vi "main.vi"() -> ()   [LabVIEW 2019]
uses:
  <instrlib>/Keithley 2600 Series/Keithley 2600 Series.lvlib
panel:
  in  "图数据":dbl[][](array[numeric])
  in  "自行输入":bool
  in  "时序优先":bool
  in  "维持时间(ms)":dbl=25.0
  in  "nplc":dbl=1.0
  in  "电压改变量":dbl=0.1 min=1e-05 max=0.1 step=1e-05
  in  "清除缓存数据":bool
  out "负时间标":timestamp
  out "正时间标":timestamp
  in  "正向状态":enum32{"SET", "RESET"}(radio)
  in  "测试人员":string
  in  "衬底":string(combo)
  in  "阻变物质":string(combo)
  in  "保存数据":bool
  out "负标记":bool
  out "正标记":bool
  out "XY图":picture
  in  "log":bool
  in  "负向扫描":bool
  in  "正向扫描":bool
  in  "反向扫描电压(V)":dbl=1.0 min=0.0 max=40.0 step=0.1
  in  "正向扫描电压(V)":dbl=1.0 min=0.0 max=40.0 step=0.1
  in  "反向极限电流(mA)":dbl=1.0 min=0.0 max=1000.0 step=0.1
  in  "正向极限电流(mA)":dbl=1.0 min=0.0 max=10.0 step=0.1
  in  "VISA resource name":refnum<visa-resource-name>
  in  "停止":bool
  in  "负":dbl[][](array[numeric])
  in  "正":dbl[][](array[numeric])
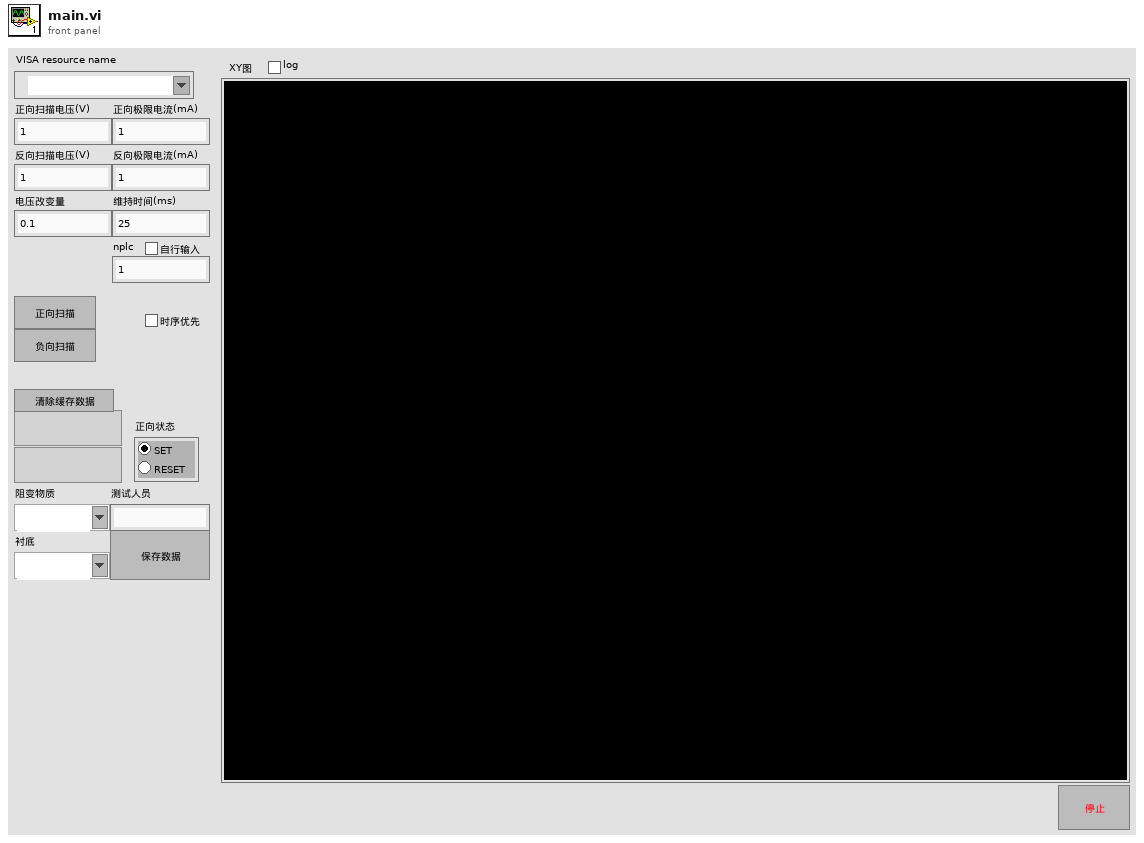
[diagram p1: front panel]
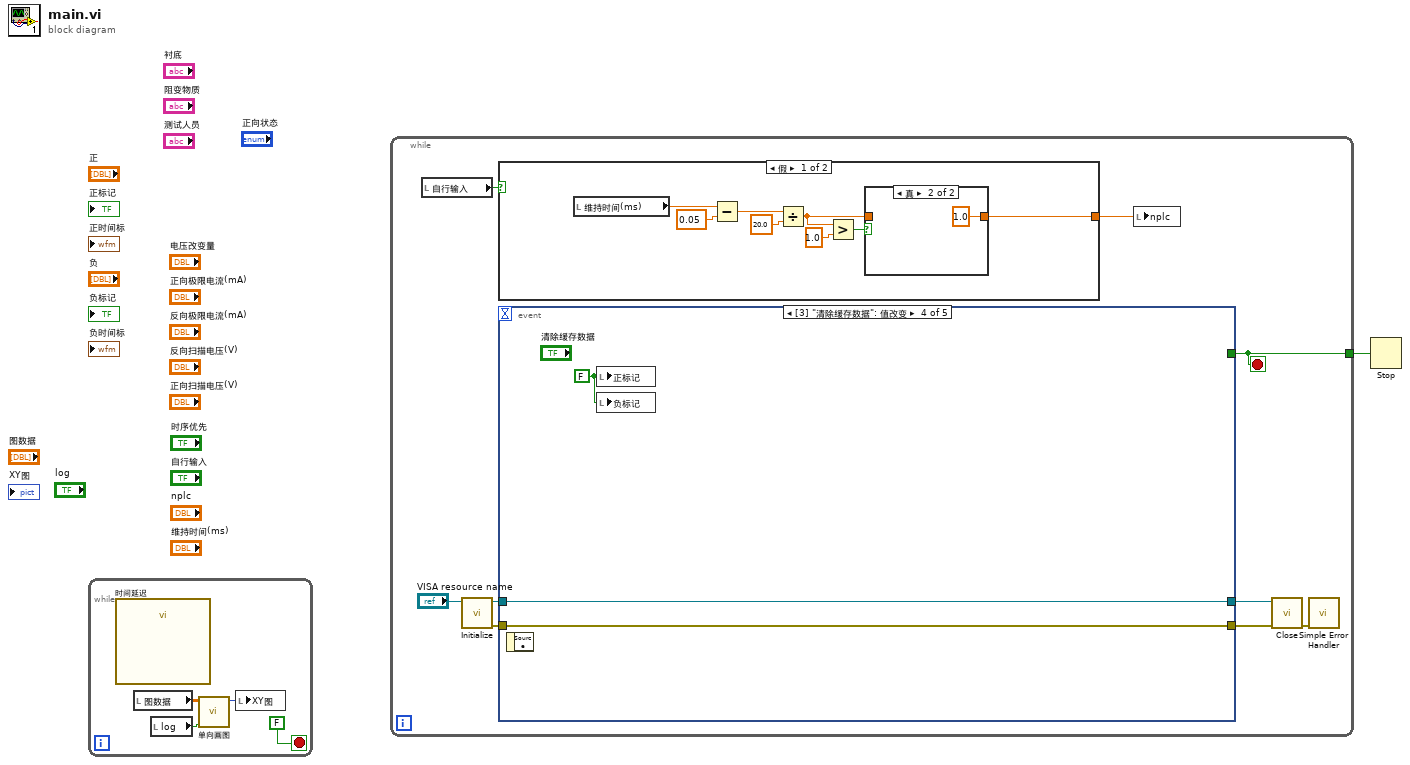
[diagram p0: block diagram]
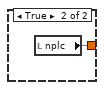
[diagram p3: hidden frame]
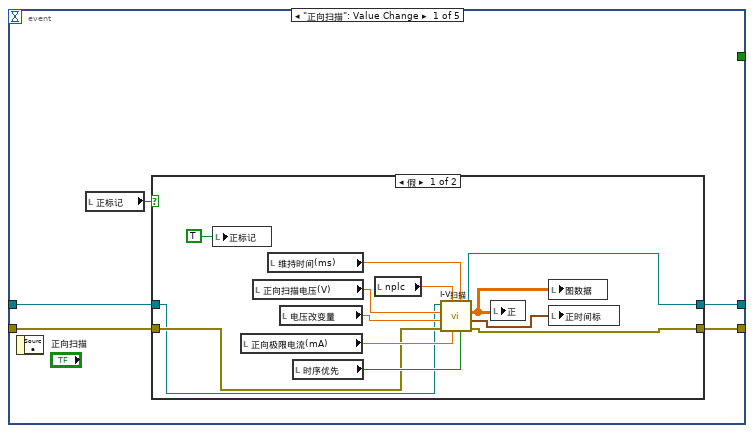
[diagram p4: hidden frame]
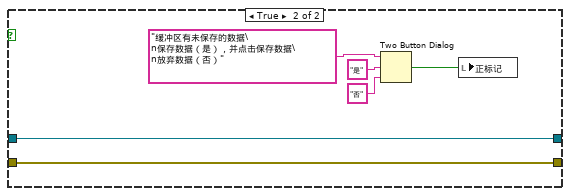
[diagram p5: hidden frame]
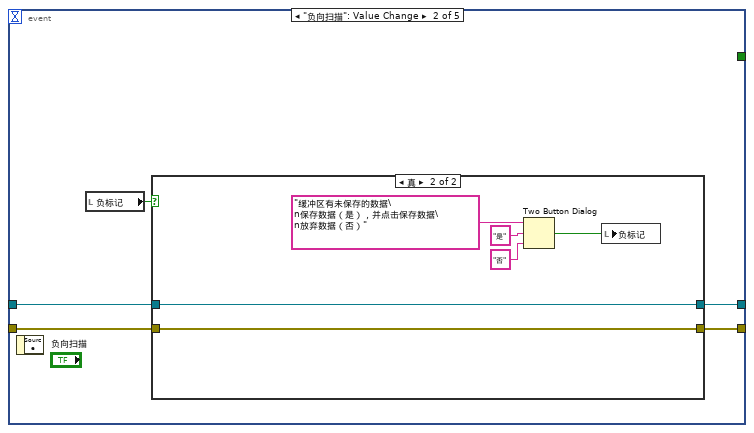
[diagram p6: hidden frame]
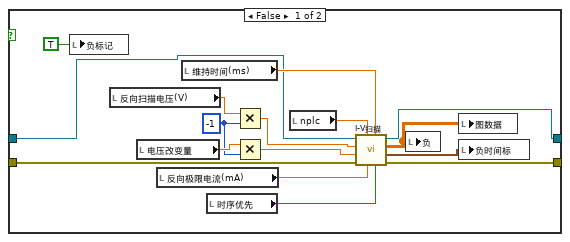
[diagram p7: hidden frame]
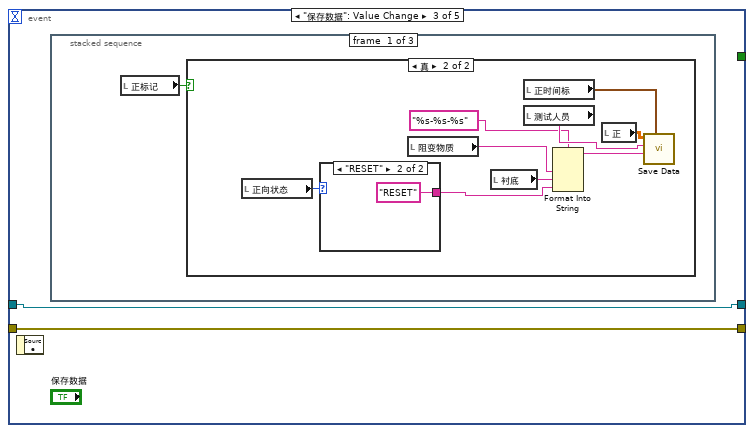
[diagram p8: hidden frame]
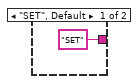
[diagram p10: hidden frame]
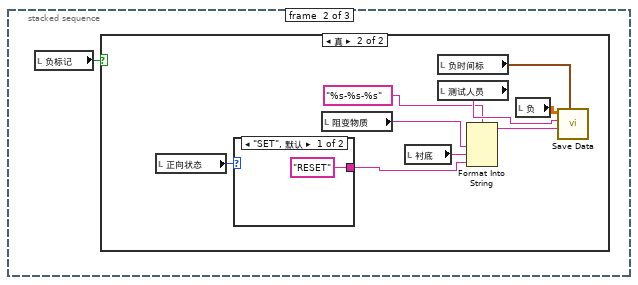
[diagram p11: hidden frame]
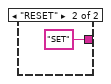
[diagram p13: hidden frame]
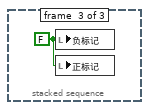
[diagram p14: hidden frame]
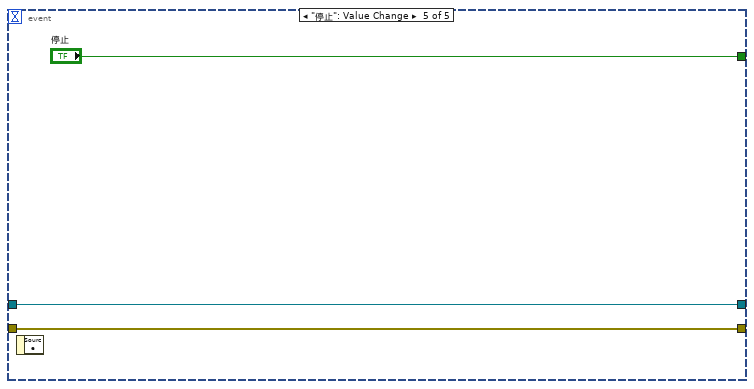
[diagram p15: hidden frame]
diagram:
  n1 = while {
    stop <- FALSE stop-if-true
    n2 = call "时间延迟"() -> ()  [unwired: 11 in, 1 out]
    n3 = local read "图数据"() -> (w4:dbl[][])
    n4 = local read "log"() -> (w3:bool)
    n5 = call "单向画图.vi"("log"=w3, "扫描数据"=w4) -> ("XY图"=w5:picture)  [unwired: 9 in]
    n6 = local write "XY图"(w5) -> ()
  }
  n7 = while {
    tunnel: [w6] -> w1
    stop <- w6 stop-if-true
    n8 = local read "自行输入"() -> (w8:bool)
    n9 = call <instrlib>:"Initialize.vi"("VISA resource name"="VISA resource name") -> ("error out"=w11:errorcluster, "VISA resource name out"=w10:refnum<visa-resource-name>)  [unwired: 9 in]
    n10 = case shown="假" w8 {
      tunnel: [w16 w25] -> w7
      frame False {
        n11 = local read "维持时间(ms)"() -> (w15:dbl)
        n12 = Subtract(x=w15, y=0.05) -> (x-y=w21:dbl)
        n13 = Divide(x=w21, y=20.0) -> (x/y=w17:dbl)
        n14 = Greater?(x=w17, y=1.0) -> (0:w18:bool)
        n15 = case shown="真" w18 {
          tunnel: w17 -> [w23 _]
          tunnel: [w23 1.0] -> w16
          frame False {
          }
          frame True {
          }
        }
      }
      frame True {
        n16 = local read "nplc"() -> (w25:dbl)
      }
    }
    n17 = event "事件结构" shown="[3] \"清除缓存数据\": 值改变" {
      selector: _ -> [_ _ _ _ _]
      dyn-events: _ -> [_ _ _ _ _]
      timeout: _ -> [_ _ _ _ _]
      tunnel: [w28 w52 w78 w106 w108] -> w12
      tunnel: [w27 w51 w77 w105 w109] -> w13
      tunnel: w11 -> [w29 w53 w77 w105 w109]
      tunnel: w10 -> [w30 w54 w78 w106 w108]
      tunnel: [_ _ _ _ "停止"] -> w6
      event "正向扫描": Value Change {
        n18 = event-data() -> ()  [unwired: 1 in, 1 out]
        n19 = local read "正标记"() -> (w26:bool)
        n20 = case shown="假" w26 {
          tunnel: w30 -> [w35 w46]
          tunnel: w29 -> [w38 w45]
          tunnel: [w33 w46] -> w28
          tunnel: [w32 w45] -> w27
          frame False {
            n21 = local write "正标记"(TRUE) -> ()
            n22 = local read "正向极限电流(mA)"() -> (w40:dbl)
            n23 = local read "正向扫描电压(V)"() -> (w36:dbl)
            n24 = local read "维持时间(ms)"() -> (w41:dbl)
            n25 = local read "电压改变量"() -> (w37:dbl)
            n26 = local read "时序优先"() -> (w42:bool)
            n27 = local read "nplc"() -> (w39:dbl)
            n28 = call "I-V扫描.vi"("时序优先"=w42, "时间点(ms)"=w41, "极限电流(mA)"=w40, "nplc"=w39, "错误输入"=w38, "电压改变量"=w37, "扫描电压(V)"=w36, "VISA资源名称"=w35) -> ("错误输出"=w32:errorcluster, "时间标识"=w34:timestamp, "扫描数据"=w31:dbl[][], "VISA资源名称输出"=w33:refnum<visa-resource-name>)
            n29 = local write "正"(w31) -> ()
            n30 = local write "图数据"(w31) -> ()
            n31 = local write "正时间标"(w34) -> ()
          }
          frame True {
            n32 = Two Button Dialog(message="缓冲区有未保存的数据\n保存数据（是），并点击保存数据\n放弃数据（否）" ("消息"), 1:"否" ("F按钮名称（“取消”）"), 2:"是" ("T按钮名称（“确定”）")) -> (T button?=w44:bool)
            n33 = local write "正标记"(w44) -> ()
          }
        }
      }
      event "负向扫描": Value Change {
        n34 = event-data() -> ()  [unwired: 1 in, 1 out]
        n35 = local read "负标记"() -> (w50:bool)
        n36 = case shown="真" w50 {
          tunnel: w54 -> [w59 w73]
          tunnel: w53 -> [w62 w72]
          tunnel: [w57 w73] -> w52
          tunnel: [w56 w72] -> w51
          frame False {
            w68 = -1
            n37 = local write "负标记"(TRUE) -> ()
            n38 = local read "反向扫描电压(V)"() -> (w70:dbl)
            n39 = local read "电压改变量"() -> (w69:dbl)
            n40 = local read "反向极限电流(mA)"() -> (w64:dbl)
            n41 = local read "维持时间(ms)"() -> (w65:dbl)
            n42 = local read "时序优先"() -> (w66:bool)
            n43 = Multiply(x=w70, y=w68) -> (x*y=w60:dbl)
            n44 = Multiply(x=w69, y=w68) -> (x*y=w61:dbl)
            n45 = local read "nplc"() -> (w63:dbl)
            n46 = call "I-V扫描.vi"("时序优先"=w66, "时间点(ms)"=w65, "极限电流(mA)"=w64, "nplc"=w63, "错误输入"=w62, "电压改变量"=w61, "扫描电压(V)"=w60, "VISA资源名称"=w59) -> ("错误输出"=w56:errorcluster, "时间标识"=w58:timestamp, "扫描数据"=w55:dbl[][], "VISA资源名称输出"=w57:refnum<visa-resource-name>)
            n47 = local write "负"(w55) -> ()
            n48 = local write "图数据"(w55) -> ()
            n49 = local write "负时间标"(w58) -> ()
          }
          frame True {
            n50 = Two Button Dialog(message="缓冲区有未保存的数据\n保存数据（是），并点击保存数据\n放弃数据（否）" ("消息"), 1:"否" ("F按钮名称（“取消”）"), 2:"是" ("T按钮名称（“确定”）")) -> (T button?=w71:bool)
            n51 = local write "负标记"(w71) -> ()
          }
        }
      }
      event "保存数据": Value Change {
        n52 = event-data() -> ()  [unwired: 1 in, 1 out]
        n53 = stacked-sequence {
          frame #0 {
            n54 = local read "正标记"() -> (w79:bool)
            n55 = case shown="真" w79 {
              frame False {
              }
              frame True {
                n56 = local read "正向状态"() -> (w84:enum32{"SET", "RESET"})
                n57 = case shown="\"RESET\"" w84 {
                  tunnel: ["SET" "RESET"] -> w83
                  frame "SET", Default {
                  }
                  frame "RESET" {
                  }
                }
                n58 = local read "阻变物质"() -> (w86:string)
                n59 = local read "衬底"() -> (w85:string)
                n60 = local read "正时间标"() -> (w80:timestamp)
                n61 = local read "测试人员"() -> (w87:string)
                n62 = Format Into String(format string="%s-%s-%s" ("格式字符串"), w86, w85, w83) -> (resulting string=w82:string)  [unwired: 2 in, 1 out]
                n63 = local read "正"() -> (w88:dbl[][])
                n64 = call "Save Data.vi"("时间标识"=w80, "数据标记"=w82, "测试人员"=w87, "扫描数据"=w88) -> ()  [unwired: 8 in]
              }
            }
          }
          frame #1 {
            n65 = local read "负标记"() -> (w91:bool)
            n66 = case shown="真" w91 {
              frame False {
              }
              frame True {
                n67 = local read "正向状态"() -> (w98:enum32{"SET", "RESET"})
                n68 = case shown="\"SET\", 默认" w98 {
                  tunnel: ["RESET" "SET"] -> w95
                  frame "SET", Default {
                  }
                  frame "RESET" {
                  }
                }
                n69 = local read "阻变物质"() -> (w97:string)
                n70 = local read "衬底"() -> (w96:string)
                n71 = local read "负时间标"() -> (w92:timestamp)
                n72 = local read "测试人员"() -> (w100:string)
                n73 = Format Into String(format string="%s-%s-%s" ("格式字符串"), w97, w96, w95) -> (resulting string=w94:string)  [unwired: 2 in, 1 out]
                n74 = local read "负"() -> (w99:dbl[][])
                n75 = call "Save Data.vi"("时间标识"=w92, "数据标记"=w94, "测试人员"=w100, "扫描数据"=w99) -> ()  [unwired: 8 in]
              }
            }
          }
          frame #2 {
            w103 = FALSE
            n76 = local write "负标记"(w103) -> ()
            n77 = local write "正标记"(w103) -> ()
          }
        }
      }
      event "清除缓存数据": Value Change {
        w104 = FALSE
        n78 = event-data() -> ()  [unwired: 1 in, 1 out]
        n79 = local write "正标记"(w104) -> ()
        n80 = local write "负标记"(w104) -> ()
      }
      event "停止": Value Change {
        n81 = event-data() -> ()  [unwired: 1 in, 1 out]
      }
    }
    n82 = local write "nplc"(w7) -> ()
    n83 = call <instrlib>:"Close.vi"("error in (no error)"=w13, "VISA resource name"=w12) -> ("error out"=w14:errorcluster)  [unwired: 9 in]
    n84 = call <vilib>:"Simple Error Handler.vi"("error in (no error)"=w14) -> ()  [unwired: 4 in, 5 out]
  }
  n85 = Stop(stop? (T)=w1) -> ()
